vi "Averaging (SubVI).vi"(9 "N":i64, 10 "result string":string, 11 "VISA Refnum in":refnum<visa-resource-name>) -> (3 "Numeric":dbl)   [LabVIEW 2020]
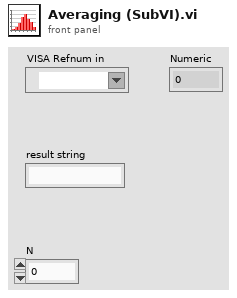
[diagram p1: front panel]
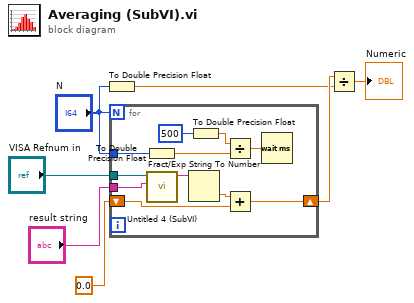
[diagram p0: block diagram]
diagram:
  n1 = To Double Precision Float(number="N") -> (double precision float=w5:dbl)
  n2 = for {
    N: "N" -> [_]
    tunnel: "N" -> [w14]
    tunnel: "result string" -> [w12]
    tunnel: "VISA Refnum in" -> [w11]
    shift-right: [w8] -> w7
    shift-left: 0.0 -> [w9]
    n3 = To Double Precision Float(number=w14) -> (double precision float=w18:dbl)
    n4 = call "Untitled 4 (SubVI).vi"("ID Query"=w12, "VISA Refnum in"=w11) -> ("read buffer"=w13:string)  [unwired: 9 in]
    n5 = Fract/Exp String To Number(string=w13) -> (number=w10:dbl)  [unwired: 3 in, 1 out]
    n6 = To Double Precision Float(number=u32 500 ("milliseconds to wait")) -> (double precision float=w17:dbl)
    n7 = Divide(x=w17, y=w18) -> (x/y=w15:dbl)
    n8 = Add(x=w10, y=w9) -> (x+y=w8:dbl)
    n9 = Wait (ms)(milliseconds to wait=w15) -> ()  [unwired: 1 out]
  }
  n10 = Divide(x=w7, y=w5) -> (x/y=→"Numeric":dbl)
